vi "Channel List Mode Init Cmd.vi"(3 "Main time":u16, 4 "Channel LF Boolean Array":bool[](array[boolean]), 5 "Channel Stim Boolean Array":bool[](array[boolean]), 6 "N factor":u8, 7 "Group Time":u8) -> (1 "Channel List Mode Init Cmd String":string)   [LabVIEW 2019]
uses:
  Bits Library/Change Bits (U8).vi
  Bits Library/Change Bit (U8).vi
  Bits Library/Bits.lvlib
panel:
  out "Checksum":u8
  out "Byte #6":u8 format="%08b"
  out "Byte #5":u8 format="%08b"
  out "Byte #4":u8 format="%08b"
  out "Byte #3":u8 format="%08b"
  out "Byte #2":u8 format="%08b"
  out "Byte #1":u8 format="%08b"
  out "Channel Stim":u8
  out "Channel LF":u8
  # "This VI implements the Channel List Mode Initialization command found on p.7 of the Hasomed RehaStim Science Mode documentation (https://issuu.com/anatomicalconcepts/docs/sciencemode_software_for_rehastim)"
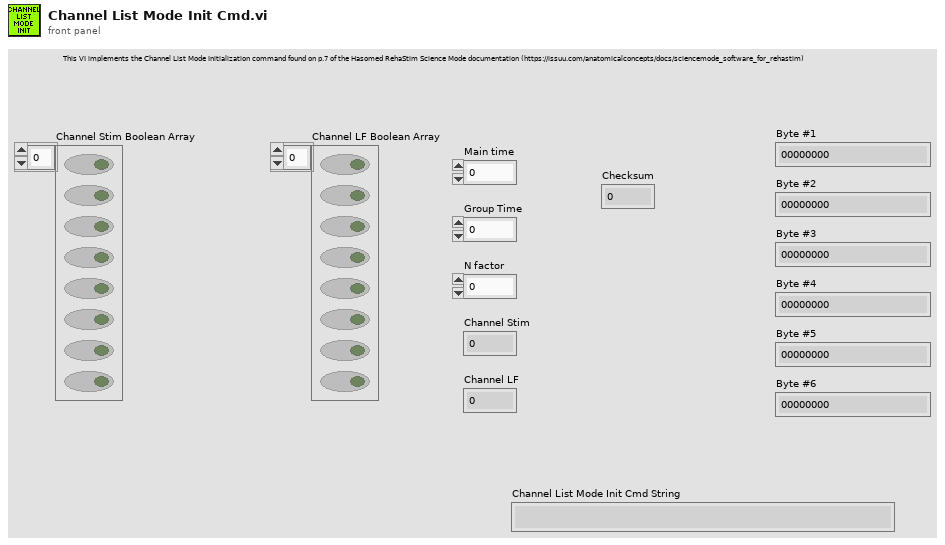
[diagram p1: front panel]
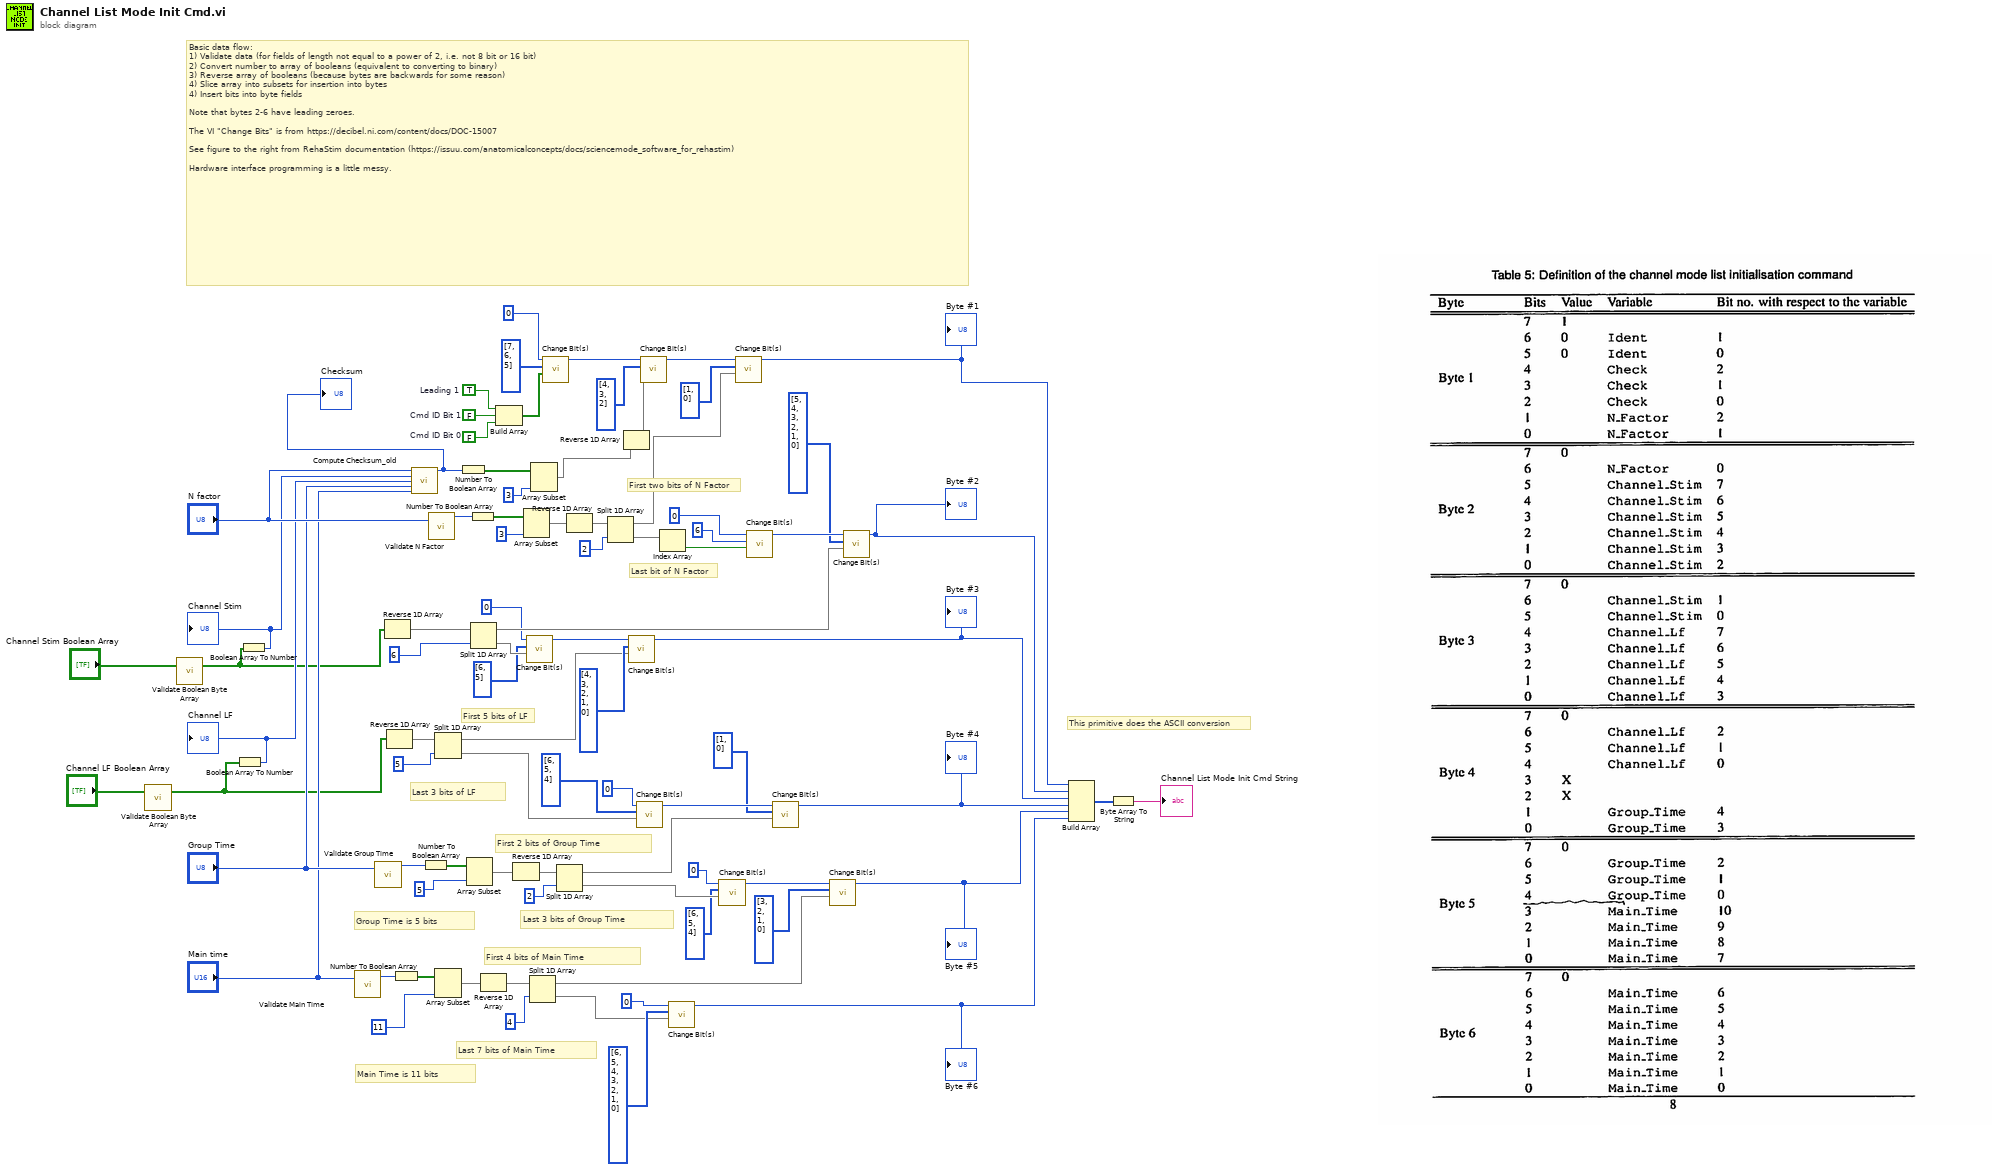
[diagram p0: block diagram]
diagram:
  w57 = FALSE  # Cmd ID Bit 0
  w58 = FALSE  # Cmd ID Bit 1
  w59 = TRUE  # Leading 1
  # "Last 7 bits of Main Time"
  # "First 4 bits of Main Time"
  # "Main Time is 11 bits"
  # "Last 3 bits of Group Time"
  # "First 2 bits of Group Time"
  # "Group Time is 5 bits"
  # "First two bits of N Factor"
  # "Last 3 bits of LF"
  # "First 5 bits of LF"
  # "This primitive does the ASCII conversion"
  # "Last bit of N Factor"
  # "Basic data flow:\n1) Validate data (for fields of length not equal to a power of 2, i.e. not 8 bit or 16 bit)\n2) Convert number to array of booleans (equivalent to converting to binary)\n3) Reverse array of booleans (because bytes are backwards for some reason)\n4) Slice array into subsets for insertion into bytes\n4) Insert bits into byte fields\n\nNote that bytes 2-6 have leading zeroes.\n\nThe VI \"Change Bits\" is from https://decibel.ni.com/content/docs/DOC-15007 \n\nSee figure to the right from RehaStim documentation (https://issuu.com/anatomicalconcepts/docs/sciencemode_software_for_rehastim) \n\nHardware interface programming is a little messy."
  n1 = call "Validate Boolean Byte Array.vi"("Channel Stim Boolean Array in"="Channel LF Boolean Array") -> ("Channel Stim Boolean Array out"=w5:bool[])  [unwired: 2 in]
  n2 = call "Validate Boolean Byte Array.vi"("Channel Stim Boolean Array in"="Channel Stim Boolean Array") -> ("Channel Stim Boolean Array out"=w7:bool[])  [unwired: 2 in]
  n3 = Boolean Array To Number(Boolean array=w5) -> (number=w9:u32)
  "Channel LF" <- w9
  n4 = Boolean Array To Number(Boolean array=w7) -> (number=w10:u32)
  "Channel Stim" <- w10
  n5 = call "Validate Main Time.vi"("Main time"="Main time") -> ("Main Time"=w41:u16)  [unwired: 2 in, 2 out]
  n6 = call "Validate Group Time.vi"("Group time"="Group Time") -> ("Group Time"=w43:u16)  [unwired: 2 in, 2 out]
  n7 = Reverse 1D Array(array=w7) -> (reversed array=w55:bool[])
  n8 = Reverse 1D Array(array=w5) -> (reversed array=w45:bool[])
  n9 = Number To Boolean Array(number=w41) -> (Boolean array=w27:bool[])
  n10 = call "Compute Checksum_old.vi"("Main time"="N factor", "Group Time"=w10, "N factor"=w9, "Channel Stim"="Group Time", "Channel LF"="Main time") -> ("Checksum"=w75:u8)  [unwired: 10 in]
  "Checksum" <- w75
  n11 = Number To Boolean Array(number=w43) -> (Boolean array=w23:bool[])
  n12 = call "Validate N Factor.vi"("N Factor"="N factor") -> ("N Factor"=w70:u8)  [unwired: 2 in, 2 out]
  n13 = Split 1D Array(array=w45, index=5) -> (first subarray=w44:bool[], second subarray=w37:bool[])
  n14 = Array Subset(array=w27, length=11) -> (w26:bool[])  [unwired: 1 in]
  n15 = Number To Boolean Array(number=w75) -> (Boolean array=w2:bool[])
  n16 = Array Subset(array=w23, length=5) -> (w22:bool[])  [unwired: 1 in]
  n17 = Number To Boolean Array(number=w70) -> (Boolean array=w68:bool[])
  n18 = Split 1D Array(array=w55, index=6) -> (first subarray=w51:bool[], second subarray=w49:bool[])
  n19 = Reverse 1D Array(array=w26) -> (reversed array=w40:bool[])
  n20 = Build Array(w59, w58, w57) -> (w56:bool[])
  n21 = Reverse 1D Array(array=w22) -> (reversed array=w42:bool[])
  n22 = Array Subset(array=w68, length=3) -> (w67:bool[])  [unwired: 1 in]
  n23 = call-poly "Change Bit(s).vi"("Values"=w49, "Bits"=i32[] [6, 5], "Number"=u8 0) -> ("Number Out"=w47:u8)  [unwired: 8 in]
  n24 = Split 1D Array(array=w40, index=4) -> (first subarray=w29:bool[], second subarray=w19:bool[])
  n25 = Array Subset(array=w2, length=3) -> (w1:bool[])  [unwired: 1 in]
  n26 = call-poly "Change Bit(s).vi"("Values"=w56, "Bits"=i32[] [7, 6, 5], "Number"=u8 0) -> ("Number Out"=w74:u8)  [unwired: 8 in]
  n27 = Split 1D Array(array=w42, index=2) -> (first subarray=w35:bool[], second subarray=w32:bool[])
  n28 = Reverse 1D Array(array=w67) -> (reversed array=w66:bool[])
  n29 = Split 1D Array(array=w66, index=2) -> (first subarray=w64:bool[], second subarray=w61:bool[])
  n30 = Reverse 1D Array(array=w1) -> (reversed array=w4:bool[])
  n31 = call-poly "Change Bit(s).vi"("Values"=w44, "Bits"=i32[] [4, 3, 2, 1, 0], "Number"=w47) -> ("Number Out"=w16:u8)  [unwired: 8 in]
  "Byte #3" <- w16
  n32 = call-poly "Change Bit(s).vi"("Values"=w37, "Bits"=i32[] [6, 5, 4], "Number"=u8 0) -> ("Number Out"=w36:u8)  [unwired: 8 in]
  n33 = call-poly "Change Bit(s).vi"("Values"=w4, "Bits"=i32[] [4, 3, 2], "Number"=w74) -> ("Number Out"=w72:u8)  [unwired: 8 in]
  n34 = Index Array(array=w61) -> (element=w60:bool)  [unwired: 1 in]
  n35 = call-poly "Change Bit(s).vi"("Values"=w19, "Bits"=i32[] [6, 5, 4, 3, 2, 1, 0], "Number"=u8 0) -> ("Number Out"=w13:u8)  [unwired: 8 in]
  "Byte #6" <- w13
  n36 = call-poly "Change Bit(s).vi"("Values"=w32, "Bits"=i32[] [6, 5, 4], "Number"=u8 0) -> ("Number Out"=w28:u8)  [unwired: 8 in]
  n37 = call-poly "Change Bit(s).vi"("Values"=w64, "Bits"=i32[] [1, 0], "Number"=w72) -> ("Number Out"=w18:u8)  [unwired: 8 in]
  "Byte #1" <- w18
  n38 = call-poly "Change Bit(s).vi"("Value"=w60, "Bit"=6, "Number"=u8 0) -> ("Number Out"=w53:u8)  [unwired: 8 in]
  n39 = call-poly "Change Bit(s).vi"("Values"=w35, "Bits"=i32[] [1, 0], "Number"=w36) -> ("Number Out"=w15:u8)  [unwired: 8 in]
  "Byte #4" <- w15
  n40 = call-poly "Change Bit(s).vi"("Values"=w29, "Bits"=i32[] [3, 2, 1, 0], "Number"=w28) -> ("Number Out"=w14:u8)  [unwired: 8 in]
  "Byte #5" <- w14
  n41 = call-poly "Change Bit(s).vi"("Values"=w51, "Bits"=u8[] [5, 4, 3, 2, 1, 0], "Number"=w53) -> ("Number Out"=w17:u8)  [unwired: 8 in]
  "Byte #2" <- w17
  n42 = Build Array(w18, w17, w16, w15, w14, w13) -> (w12:u8[])
  n43 = Byte Array To String(unsigned byte array=w12) -> (string=→"Channel List Mode Init Cmd String":string)
